vi "Read MaxFluence.vi"(8 "error in (no error)":errorcluster, 11 "Analyze Results Fluence in":refnum<class "Analyze Results Fluence.lvclass">) -> (0 "error out":errorcluster, 2 "MaxFluence":dbl[unit], 3 "Analyze Results Fluence out":refnum<class "Analyze Results Fluence.lvclass">)   [LabVIEW 2014, in "Analyze Results Fluence.lvclass"]
uses:
  Analyze Results Fluence.lvclass
  Analyze Results Fluence.lvclass/Analyze Results Fluence.ctl
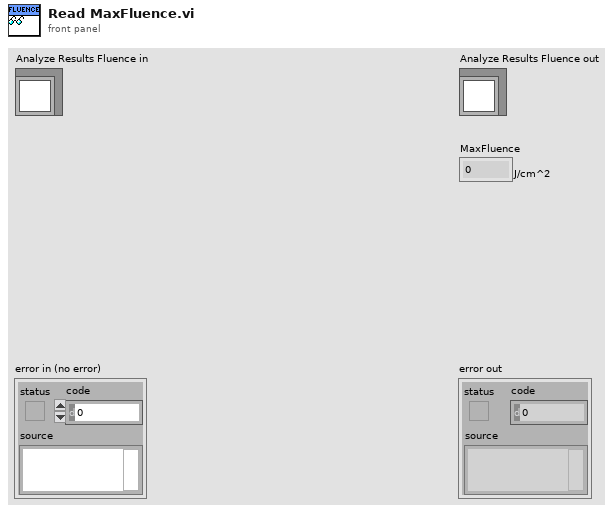
[diagram p1: front panel]
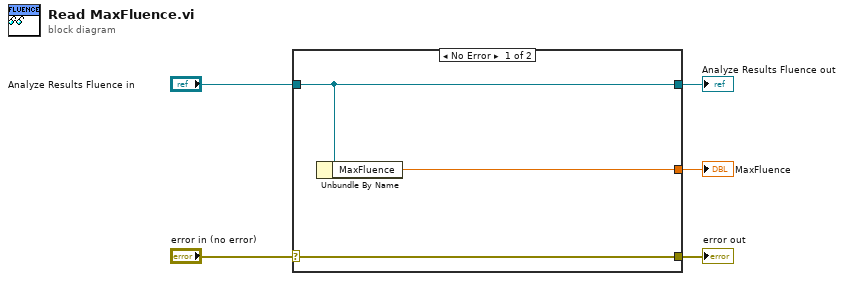
[diagram p0: block diagram]
diagram:
  n1 = case shown="No Error" "error in (no error)" {
    selector: "error in (no error)" -> [w8 w9]
    tunnel: [w8 w9] -> w4
    tunnel: [w7 w10] -> w2
    tunnel: "Analyze Results Fluence in" -> [w7 w10]
    tunnel: [w6 _] -> w1
    frame No Error {
      n2 = Unbundle By Name(w7) -> ("MaxFluence"=w6:dbl[unit])
    }
    frame Error {
    }
  }
  "error out" <- w4
  "Analyze Results Fluence out" <- w2
  "MaxFluence" <- w1
